vi "Test_ConstructTransport_InvalidRefnum_Error.vi"(8 "error in (no error)":errorcluster, 11 "TestCase in":refnum<class "TestRingStringsBinding.lvclass">) -> (0 "error out":errorcluster, 3 "TestCase out":refnum<class "TestRingStringsBinding.lvclass">)   [LabVIEW 2017, in "TestRingStringsBinding.lvclass"]
uses:
  TestRingStringsBinding.lvclass
  Source/Concrete/RingStringsBinding/RingStringsBinding.lvclass
panel:
  out "Return Error":errorcluster
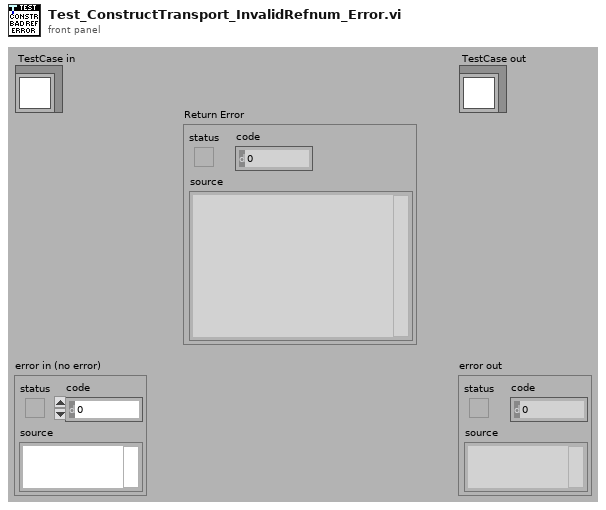
[diagram p1: front panel]
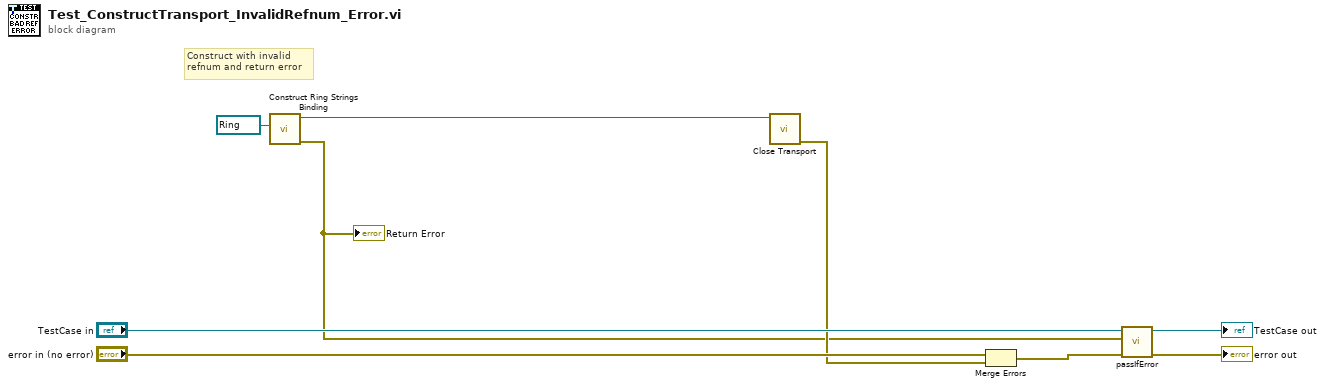
[diagram p0: block diagram]
diagram:
  # "Construct with invalid\nrefnum and return error"
  n1 = call "Construct Ring Strings Binding.vi"("Ring Refnum"=refnum<vi> refnum) -> ("error out"=w1:errorcluster, "RingStringsBinding"=w5:refnum<class "RingStringsBinding.lvclass">)  [unwired: 9 in]
  "Return Error" <- w1
  n2 = call-dynamic "Close Transport.vi"("ITransport in"=w5) -> ("error out"=w3:errorcluster)  [unwired: 10 in]
  n3 = Merge Errors("error in (no error)", w3) -> (w4:errorcluster)
  n4 = call-dynamic "passIfError.vi"("error in (no error)"=w4, "error"=w1, "TestCase in"="TestCase in") -> ("error out"=→"error out":errorcluster, "TestCase out"=→"TestCase out":refnum<class "TestRingStringsBinding.lvclass">)  [unwired: 7 in]
